vi "Pre Launch Init.vi"(11 "GUI Actor in":refnum<class "GUI Actor.lvclass">) -> (0 "error out":errorcluster, 3 "GUI Actor out":refnum<class "GUI Actor.lvclass">)   [LabVIEW 2020, in "GUI Actor.lvlib" / "GUI Actor.lvclass"]
doc: "(<B>Filename</B>: Actor Framework.lvlib:Actor.lvclass:Pre Launch Init.vi)\n\nDefines behavior that occurs after the Launch Nested Actor method is invoked but before the actor's Actor Core method begins running.\n\nBy default, this method does nothing. A descendant class may override it to define behavior."
uses:
  GUI Actor.lvclass
  <vilib>/ActorFramework/Actor/Actor.lvclass
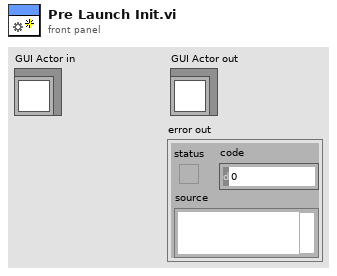
[diagram p1: front panel]
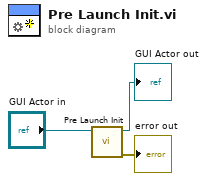
[diagram p0: block diagram]
diagram:
  n1 = call-parent "Pre Launch Init.vi"("Actor in"="GUI Actor in") -> ("error out"=→"error out":errorcluster, "Actor out"=→"GUI Actor out":refnum<class "GUI Actor.lvclass">)  [unwired: 9 in]
